vi "FGV Map Delete Instance.vi"(8 "error in (no error)":errorcluster, 11 "Instance Key":string) -> (0 "error out":errorcluster, 2 "Instance Not Found ?":bool, 3 "Deleted Instance":map{string, variant}(c390))   [LabVIEW 2020, in "FGV Map.lvlib"]
uses:
  FGV Map.lvlib
  Controls/FGV Map Core State.ctl
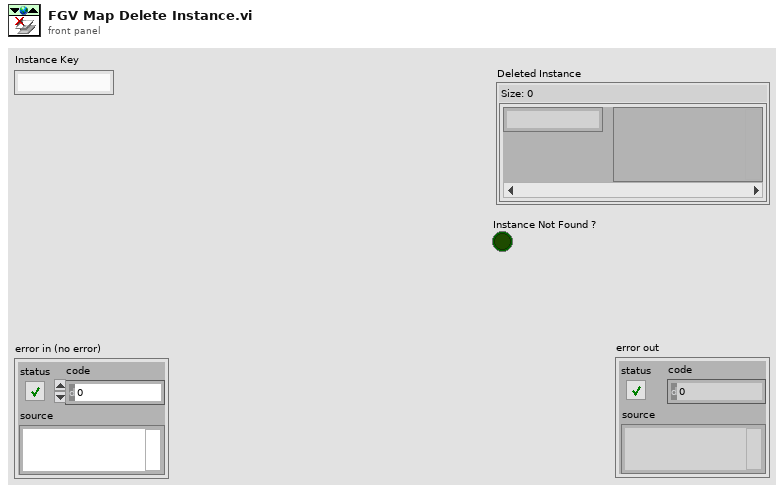
[diagram p1: front panel]
types:
  T1 = typedef "FGV Map.lvlib/FGV Map Core State.ctl" = enum16{"Init", "Set Instance (Unlock)", "Get Instance", "Get Instance (Lock)", "Unlock", "Get All Instances", "Delete Instance"}
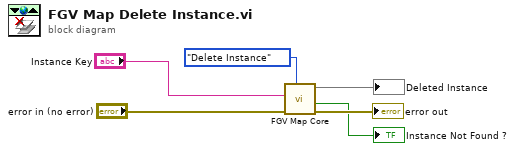
[diagram p0: block diagram]
diagram:
  n1 = call "FGV Map Core.vi"("FGV State"=FGV_Map_Core_State."Delete Instance", "error in"="error in (no error)", "Instance Key"="Instance Key") -> ("error out"=→"error out":errorcluster, "Instance Not Found ?"=→"Instance Not Found ?":bool, "Instance Out"=→"Deleted Instance":map{string, variant})  [unwired: 4 in, 2 out]
